vi "Read Filepath.vi"(11 "SQLite Database in":refnum<class "SQLite Database.lvclass">) -> (2 "File Path Indicator":path, 3 "SQLite Database out":refnum<class "SQLite Database.lvclass">)   [LabVIEW 2019, in "TSC Event Logger.lvlib" / "SQLite Database.lvclass"]
doc: "Read the filepath to the database sink."
uses:
  SQLite Database.lvclass
  SQLite Database.lvclass/SQLite Database.ctl
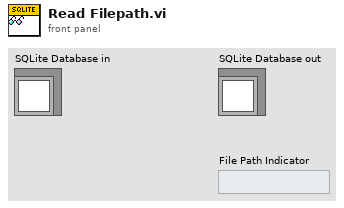
[diagram p1: front panel]
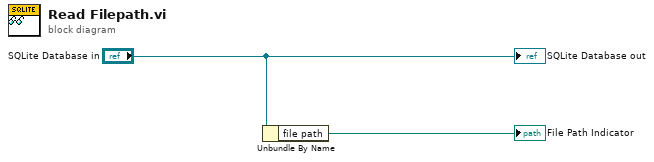
[diagram p0: block diagram]
diagram:
  n1 = Unbundle By Name("SQLite Database in") -> ("file path"=→"File Path Indicator":path)
  "SQLite Database out" <- "SQLite Database in"
